vi "Trav_3D_volume.vi"(3 "Simulate/Run":T1, 5 "multirunIn":T2={"Start X"=0.0, "Start Y"=0.0, "Start Z"=0.0, "End X"=0.0, "End Y"=0.0, "End Z"=0.0, "nPoints"=0, "Spacing"=enum."Linear", "Filename"=path "", "Tunnel Speed"=0.0, "Averaging time (mins)"=0.0, "Extra Commands"="", "Carrier_1 Q (l/min)"=0.0, "Carrier_2 Q (l/min)"=0.0, "Trace Gas Concentration (%)"=0.0, "Specific Arguments"="", "Comments"="", "Row No"=0, "Row Type Selector"=enum."Traverse 3D Volume", "EstCompl"="", "Row Duration (mins)"=0.0, "nValidPoints"=0, "Meas Setup File"=""} {"Carrier_2 Q (l/min)" format="%#.2f"; "Row Duration (mins)" format="%#.1f"; "Row No" min=0; "Trace Gas Concentration (%)" min=0.0 format="%#_4f"; "Carrier_1 Q (l/min)" format="%#.4f"; "Start X" format="%#.2f"; "Start Y" format="%#.2f"; "Start Z" format="%#.2f"; "End X" format="%#.2f"; "End Y" format="%#.2f"; "End Z" format="%#.2f"; "Tunnel Speed" format="%#.2f"; "Averaging time (mins)" min=0.0 format="%#.2f"}) -> (0 "Error Messages":string, 1 "Status":T5, 2 "multirunOut":T2 {"Carrier_2 Q (l/min)" format="%#.2f"; "Row Duration (mins)" format="%#.1f"; "Row No" min=0; "Trace Gas Concentration (%)" min=0.0 format="%#_4f"; "Carrier_1 Q (l/min)" format="%#.4f"; "Start X" format="%#.2f"; "Start Y" format="%#.2f"; "Start Z" format="%#.2f"; "End X" format="%#.2f"; "End Y" format="%#.2f"; "End Z" format="%#.2f"; "Tunnel Speed" format="%#.2f"; "Averaging time (mins)" min=0.0 format="%#.2f"})   [LabVIEW 2021]
uses:
  Globals/Trav_pos_global.vi
  Globals/Meas_global.vi
  Controls/User_Specific_mode.ctl
  Gen Trav/Multi_Run_Status.ctl
  Controls/Setup.ctl
  Controls/Save_Data.ctl
  Controls/Overhead.ctl
  ADAM Client/Sub VIs/ADAM Controls/Traverse_Level_State.ctl
  Globals/Preference_global.vi
  Gen Trav/Spacing.ctl
  Gen Trav/Traverse_cluster.ctl
  Controls/Multi_run_mode.ctl
panel:
  in  "moveCostWeighting":sgl[](array[numeric])=[5.0, 2.0, 1.0]
  out "PredictedEnd":timestamp format="%<%H:%M\n%a %d>T"
  out "StartTime":timestamp format="%<%H:%M\n%a %d>T"
  out "Progress":i32(slide) scale=0.0..20.0
  in  "pointIDs":string[](array[string])
  in  "pointComments":string[](array[string])
  out "Pause message":string
  in  "Pause":bool
  out "Current position":dbl[](array[numeric]) format="%.2f"
  in  "stop":bool
  in  "Array of Positions":dbl[][](array[numeric]) format="%.2f"
  out "Abcissa copy":string="Y (mm)"
  out "Abcissa":string="Y (mm)"
  in  "Plot 1":i32[](listbox)=[1]
  out "U":cluster{dbl[], dbl[]}[](graph)
  out "% u'/U":cluster{dbl[], dbl[]}[](graph)
  # "Current Point"
  # "X           Y          Z"
  # "Start"
  # "End"
  # "X           Y          Z"
  # "Start"
  # "End"
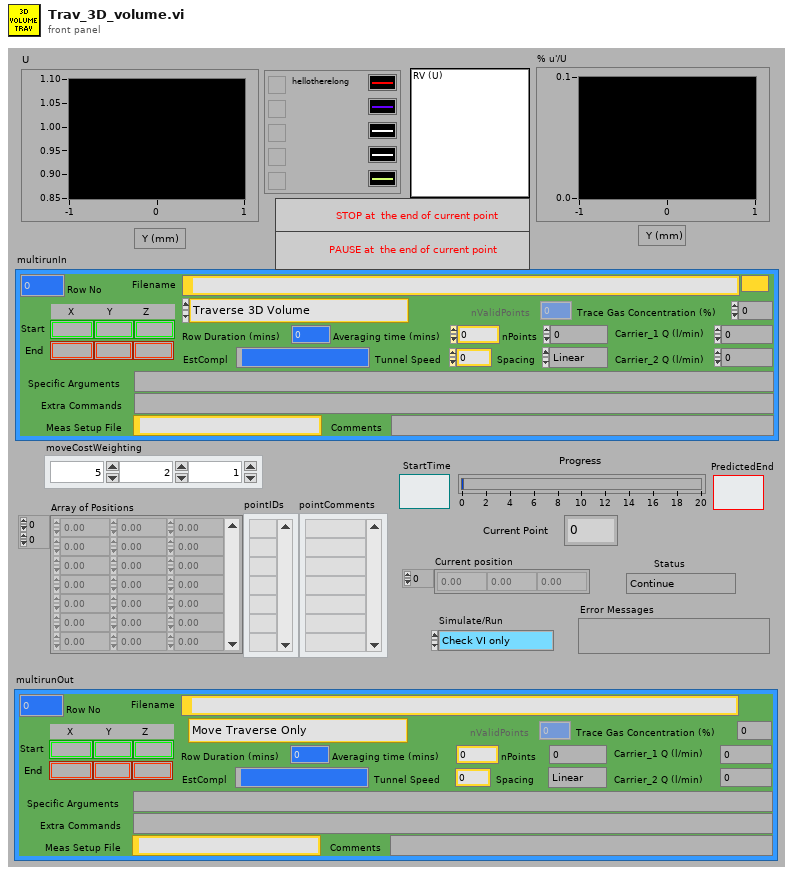
[diagram p1: front panel]
types:
  T1 = typedef "User_Specific_mode.ctl" = enum16{"Check VI only", "Run VI"}
  T2 = typedef "Traverse_cluster.ctl" = cluster{"Start X":sgl, "Start Y":sgl, "Start Z":sgl, "End X":sgl, "End Y":sgl, "End Z":sgl, "nPoints":i32, "Spacing":T3, "Filename":path, "Tunnel Speed":dbl, "Averaging time (mins)":dbl, "Extra Commands":string, "Carrier_1 Q (l/min)":dbl, "Carrier_2 Q (l/min)":dbl, "Trace Gas Concentration (%)":dbl, "Specific Arguments":string, "Comments":string, "Row No":i32, "Row Type Selector":T4, "EstCompl":string, "Row Duration (mins)":dbl, "nValidPoints":i32, "Meas Setup File":string}
  T3 = typedef "Spacing.ctl" = enum16{"Linear", "Log", "Gauss", "Specified", "N/A"}
  T4 = typedef "Multi_run_mode.ctl" = enum16{"Move Traverse Only", "Set Tunnel Speed Only", "Set Source Only", "Set Measurement Conditions", "Single Measurement", "Vertical Profile", "Lateral Profile", "Longitudinal Profile", "Multi-Axis Profile", "Explore Volume", "Auto Calibrate", "Meas Fast FID Bkgnd", "Check Beam Power", "Scanning Valve Measurement", "Run VI Named:", "Set ADAM Ch", "Wait (minutes)", "Send Message", "Synchronize With:", "Fall Back to this Row", "Turn Off Row Repeating", "Traverse 3D Volume", "Blank Row", "Jump to Fall Back Row"}
  T5 = typedef "Multi_Run_Status.ctl" = enum16{"Continue", "Continue with Error", "Jump to Next Point", "Jump to Next Row", "Jump To Fall Back", "Terminate Run"}
  T6 = typedef "Overhead.ctl" = enum16{"Update total times", "Read Current Overhead", "Re Scale totals to 3 hrs", "Initialise totals to 3hr"}
  T7 = typedef "Save_Data.ctl" = enum16{"Save No Data", "Save Data"}
  T8 = typedef "Setup.ctl" = enum16{"Run Program", "Show Setup", "Save Current Setup", "Setup Front Panel"}
  T9 = typedef "Traverse_Level_State.ctl" = enum16{"Running", "Complete"}
  T10 = typedef "GMU Gas Line Name.ctl" = enum16{"GMU1 Source", "GMU2 Source", "GMU2 Calib", "CPP GRC-A", "CPP GRC-B"}
  T11 = typedef "Status_Cluster.ctl" = cluster{"Status":T5, "Error Type":string, "Error Description":string}
  T12 = typedef "Analysis_info_cluster.ctl" = cluster{"Colour":u32, "Inst type":T13, "Inst name":string, "Symbol":string, "Code name":string, "Extra Info":string, "Inst Array":T14, "Extra Titles":string[], "Extra Values":string[], "U":dbl, "u^2":dbl, "u^3":dbl, "u^4":dbl, "Skew_u":dbl, "Kurt_u":dbl, "Sd Error in Mean":dbl, "% u'/U":dbl, "X":dbl, "Y":dbl, "Z":dbl, "Timescale integral Estimate":dbl, "Sd Error in Variance":dbl, "Calib File":path, "Calib Constants":dbl[], "Output Position":bool, "Stats":enum16{"None", "Basic", "Full"}, "Av Sampling Rate":dbl, "Av No of Samples":dbl, "Total Meas Time (s)":dbl, "ADAM Ch Name":string, "Max value":dbl, "Min value":dbl, "Req Sample Rate Hz":dbl, "Sync Delay Time (s)":dbl, "Ch No":i16, "Device":string, "Use Latest Calib":bool, "Port":string, "Metadata Ch Names":string[], "Metadata Ch Values":string[], "Label":string}
  T13 = typedef "Inst_type.ctl" = enum16{"Raw voltage", "Raw with zero offsetting", "Propeller anemometer", "Pressure Transducer", "Pitot-static tube", "Hot wire", "Cross wire 1", "Cross wire 2", "Generic Linear", "Generic Polynomial", "Generic BackPoly", "Fast FID", "Thermocouple", "Cold wire", "Pulsed Wire", "LDA Vel", "LDA Tran time", "LDA Arr time", "Microphone"}
  T14 = typedef "Instrument_Array.ctl" = enum16{"PWA", "LDA", "Analogue"}
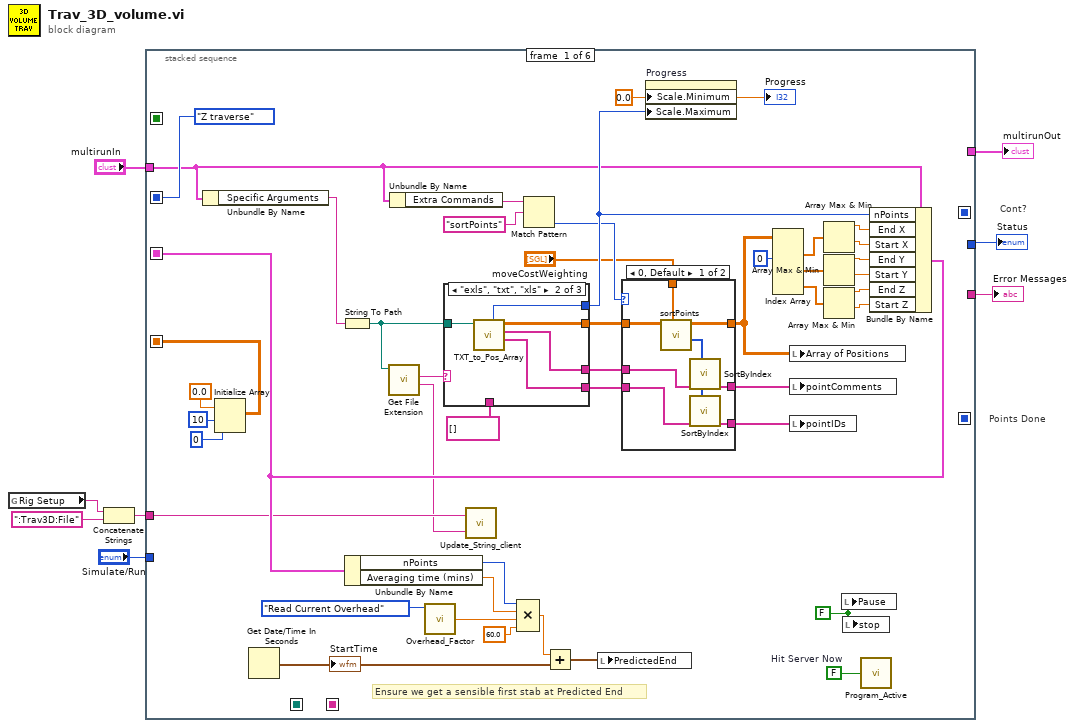
[diagram p0: block diagram]
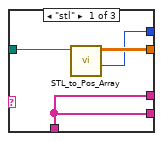
[diagram p3: hidden frame]
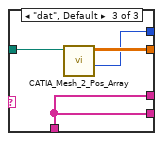
[diagram p4: hidden frame]
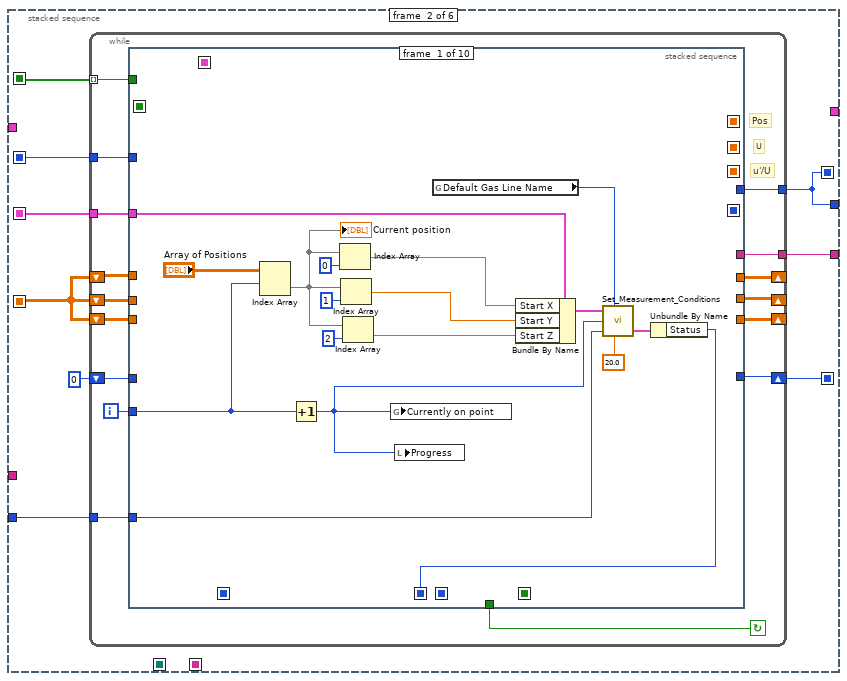
[diagram p5: hidden frame]
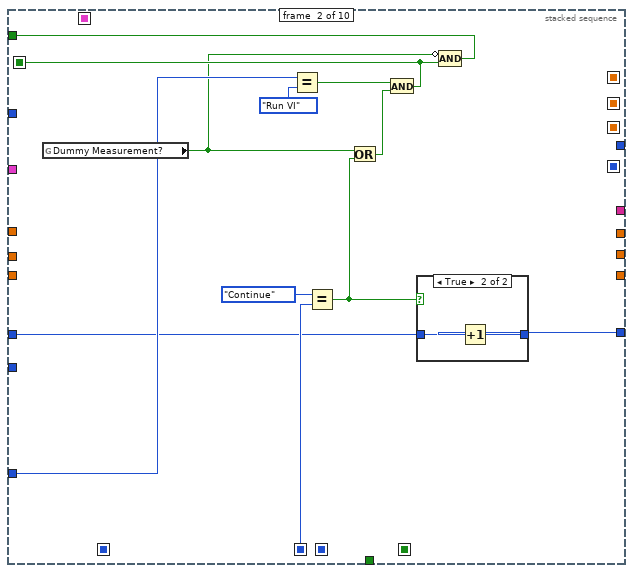
[diagram p6: hidden frame]
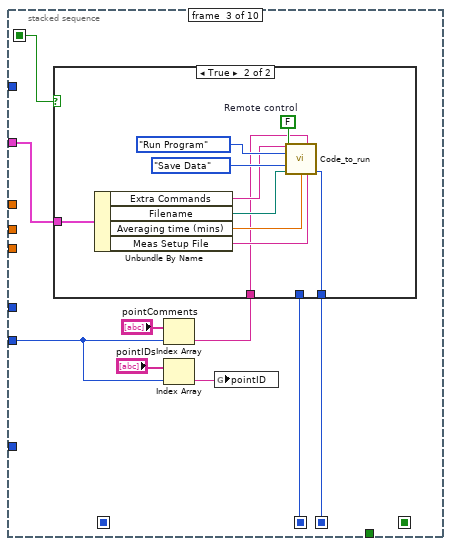
[diagram p8: hidden frame]
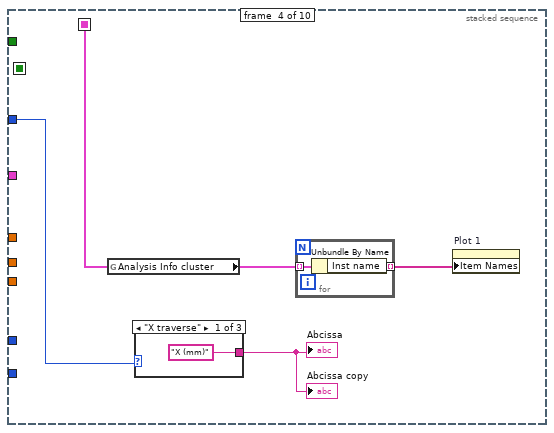
[diagram p10: hidden frame]
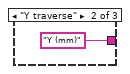
[diagram p11: hidden frame]
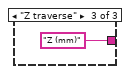
[diagram p12: hidden frame]
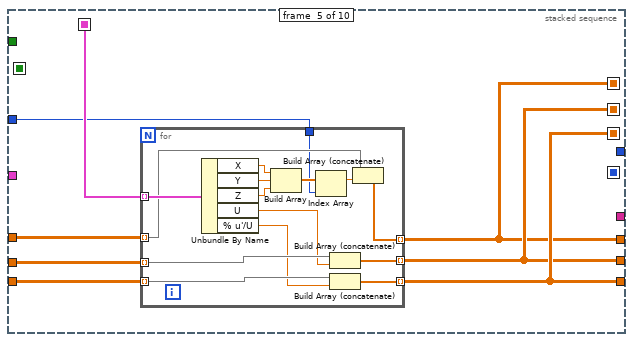
[diagram p13: hidden frame]
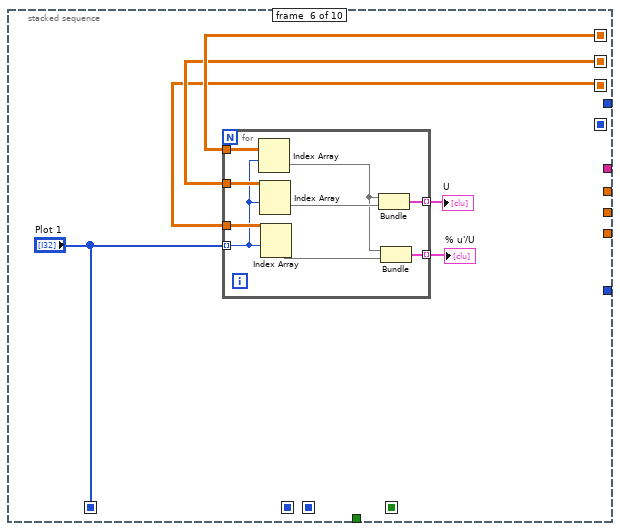
[diagram p14: hidden frame]
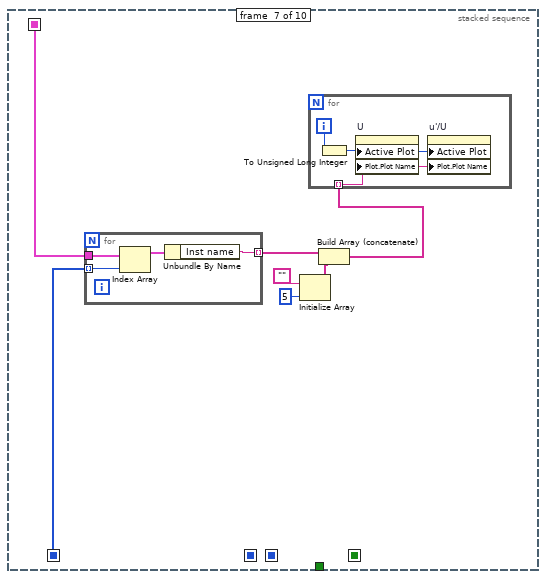
[diagram p15: hidden frame]
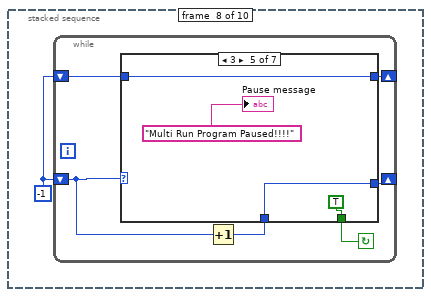
[diagram p16: hidden frame]
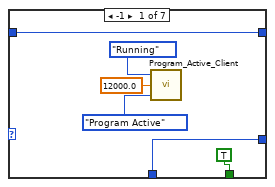
[diagram p17: hidden frame]
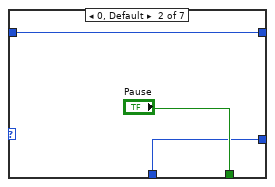
[diagram p18: hidden frame]
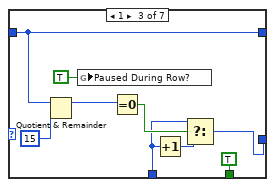
[diagram p19: hidden frame]
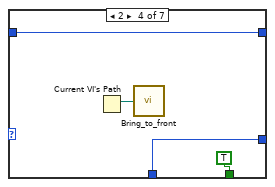
[diagram p20: hidden frame]
diagram:
  # "Points Done"
  # "Cont?"
  n1 = global read "Preference_global.vi" "Rig Setup"() -> (w4:string)
  n2 = Concatenate Strings(w4, ":Trav3D:File" ("string")) -> (w2:string)
  n3 = stacked-sequence {
    seq-local: [w50 _ _ _ _ _] -> [_ w85 _ _ _ _]
    seq-local: [enum16{"X traverse", "Y traverse", "Z traverse"}."Z traverse" ("Axis Traversed") _ _ _ _ _] -> [_ w86 _ _ _ _]
    seq-local: [_ _ w330 _ _ _] -> [_ _ _ _ w354 _]
    seq-local: [_ _ _ w337 _ _] -> [_ _ _ _ w353 _]
    seq-local: [_ w84 _ _ _ _] -> [_ _ _ _ _ _]
    seq-local: [_ w82 _ _ _ _] -> [_ _ _ w334 w352 _]
    seq-local: [_ w80 _ _ _ _] -> [_ _ _ _ _ w361]
    seq-local: [w30 _ _ _ _ _] -> [_ w79 _ _ _ w363]
    tunnel: [_ w84 _ _ _ _] -> w6
    tunnel: [_ _ _ _ _ w373] -> w8
    tunnel: "Simulate/Run" -> [_ w83 _ _ _ w372]
    tunnel: [_ w78 _ _ _ _] -> w5
    tunnel: w2 -> [w14 _ _ _ _ w360]
    tunnel: "multirunIn" -> [w10 _ _ _ _ _]
    frame #0 {
      w33 = 0.0 ("Data Entry Limits:Minimum")
      w48 = FALSE ("stop")
      w49 = FALSE  # Hit Server Now
      # "Ensure we get a sensible first stab at Predicted End"
      n4 = Unbundle By Name(w10) -> ("Specific Arguments"=w46:string)
      n5 = Initialize Array(0.0, 10, 0) -> (w50:dbl[][])
      n6 = Get Date/Time In Seconds() -> (seconds since 1Jan1904=w31:timestamp)
      "StartTime" <- w31
      n7 = String To Path(string=w46) -> (path=w13:path)
      n8 = call <vilib>:"Get File Extension.vi"("file"=w13) -> ("filename without extension"=w12:string, "lowercase file extension"=w11:string)  [unwired: 6 in, 3 out]
      n9 = Unbundle By Name(w10) -> ("Extra Commands"=w17:string)
      n10 = call "Overhead_Factor.vi"("Mode"=Overhead."Read Current Overhead") -> ("Current Overhead Factor"=w27:dbl)  [unwired: 3 in]
      n11 = case shown="\"exls\", \"txt\", \"xls\"" w11 {
        tunnel: [w67 w72 w77] -> w23
        tunnel: [w66 w70 w76] -> w34
        tunnel: w13 -> [w68 w73 w75]
        tunnel: [w65 w71 w74] -> w21
        tunnel: string[] [] ("pointComments") -> [w65 _ w74]
        tunnel: [w65 w69 w74] -> w19
        frame "stl" {
          n12 = call "STL_to_Pos_Array.vi"("STL file"=w68) -> ("Number of Points"=w66:i32, "Array of Positions"=w67:dbl[][])  [unwired: 9 in]
        }
        frame "exls", "txt", "xls" {
          n13 = call "TXT_to_Pos_Array.vi"("pointfile"=w73) -> ("pointIDs"=w69:string[], "pointComments"=w71:string[], "pointsXYZArray"=w72:dbl[][], "Number of Points"=w70:i32)  [unwired: 5 in, 2 out]
        }
        frame "dat", Default {
          n14 = call "CATIA_Mesh_2_Pos_Array.vi"("Catia Mesh File"=w75) -> ("Number of Points"=w76:i32, "Array of Positions"=w77:dbl[][])  [unwired: 9 in]
        }
      }
      n15 = call "Update_String_client.vi"("String"=w12, "Ch Name"=w14) -> ()  [unwired: 1 in]
      n16 = Match Pattern(string=w17, regular expression="sortPoints") -> (offset past match=w15:i32)  [unwired: 1 in, 3 out]
      n17 = case shown="0, Default" w15 {
        tunnel: w23 -> [w61 w64]
        tunnel: [w60 w64] -> w22
        tunnel: w21 -> [w59 w63]
        tunnel: [w58 w63] -> w20
        tunnel: w19 -> [w57 w62]
        tunnel: [w56 w62] -> w18
        tunnel: "moveCostWeighting" -> [w54 _]
        frame 0, Default {
          n18 = call "sortPoints.vi"("moveCostWeighting"=w54, "targetCoords"=w61) -> ("sortOrder"=w55:i32[], "sortedCoords"=w60:sgl[][])  [unwired: 8 in]
          n19 = call "SortByIndex.vi"("sortOrder"=w55, "1DstringIn"=w59) -> ("1DstringOut"=w58:string[])  [unwired: 4 in, 2 out]
          n20 = call "SortByIndex.vi"("sortOrder"=w55, "1DstringIn"=w57) -> ("1DstringOut"=w56:string[])  [unwired: 4 in, 2 out]
        }
        frame -1 {
        }
      }
      n21 = property on="Progress" class="Slide (strict)"("Scale.Minimum"=w33, "Scale.Maximum"=w34) -> ()  [unwired: 2 in, 2 out]
      n22 = Index Array(array=w22, index (col) #1=0 ("disabled index (col)")) -> (element #1=w43:dbl[], element #2=w40:dbl[], element #3=w35:dbl[])  [unwired: 5 in]
      n23 = local write "Array of Positions"(w22) -> ()
      n24 = local write "pointComments"(w20) -> ()
      n25 = local write "pointIDs"(w18) -> ()
      n26 = Array Max & Min(array=w43) -> (max value=w42:dbl, min value=w41:dbl)  [unwired: 2 out]
      n27 = Array Max & Min(array=w40) -> (max value=w39:dbl, min value=w38:dbl)  [unwired: 2 out]
      n28 = Array Max & Min(array=w35) -> (max value=w37:dbl, min value=w36:dbl)  [unwired: 2 out]
      n29 = local write "Pause"(w48) -> ()
      n30 = local write "stop"(w48) -> ()
      n31 = call "Program_Active.vi"("Hit Server Now"=w49) -> ()
      n32 = Bundle By Name(cluster=w10, "nPoints"=w34, "End X"=w42, "Start X"=w41, "End Y"=w39, "Start Y"=w38, "End Z"=w37, "Start Z"=w36) -> (w30:T2)
      n33 = Unbundle By Name(w30) -> ("nPoints"=w29:i32, "Averaging time (mins)"=w28:dbl)
      n34 = Compound Arithmetic op=MULTIPLY(w29, w28, w27, 60.0 ("value")) -> (w26:dbl)
      n35 = Add(x=w26, y=w31) -> (x+y=w25:timestamp)
      n36 = local write "PredictedEnd"(w25) -> ()
      "Progress" <- w33
    }
    frame #1 {
      n37 = while {
        shift-left: 0 -> [w89]
        shift-right: [w88] -> w80
        tunnel: [w90] -> w82 mode=indexing
        tunnel: w79 -> [w91]
        tunnel: w83 -> [w92]
        tunnel: [w93] -> w84
        shift-left: w85 -> [w96]
        shift-right: [w95] -> _
        tunnel: w86 -> [w97]
        shift-left: w85 -> [w99]
        shift-right: [w98] -> _
        shift-left: w85 -> [w101]
        shift-right: [w100] -> _
        tunnel: [w87] -> w78
        i -> [w102]
        stop <- w94 continue-if-true
        # "Pos"
        # "U"
        # "u'/U"
        n38 = stacked-sequence {
          seq-local: [_ _ _ w158 _ _ _ _ _ _] -> [_ _ _ _ w169 _ w202 _ _ _]
          seq-local: [_ _ _ _ w165 _ _ _ _ _] -> [_ _ _ _ _ w192 _ _ _ _]
          seq-local: [_ _ _ _ w167 _ _ _ _ _] -> [_ _ _ _ _ w191 _ _ _ _]
          seq-local: [_ _ _ _ w168 _ _ _ _ _] -> [_ _ _ _ _ w190 _ _ _ _]
          seq-local: [_ _ _ _ _ "Plot 1" _ _ _ _] -> [_ _ _ _ _ _ w208 _ _ _]
          seq-local: [_ _ w142 _ _ _ _ _ _ _] -> [_ _ _ _ _ _ _ _ w266 _]
          seq-local: [w109 _ _ _ _ _ _ _ _ _] -> [_ w129 w140 _ _ _ _ _ _ _]
          seq-local: [_ w122 _ _ _ _ _ _ _ _] -> [_ _ w141 _ _ _ _ _ _ _]
          seq-local: [_ _ _ _ _ _ _ _ w261 _] -> [_ _ _ _ _ _ _ _ _ w283]
          seq-local: [_ _ _ _ _ _ _ _ w260 _] -> [_ _ _ _ _ _ _ _ _ w277]
          tunnel: w102 -> [w107 _ w136 _ _ _ _ _ w272 w280]
          tunnel: w101 -> [_ _ _ _ w171 _ _ _ _ _]
          tunnel: [_ _ _ _ w167 _ _ _ _ _] -> w100
          tunnel: w99 -> [_ _ _ _ w170 _ _ _ _ _]
          tunnel: [_ _ _ _ w168 _ _ _ _ _] -> w98
          tunnel: w97 -> [_ _ _ w156 w164 _ _ _ _ _]
          tunnel: w96 -> [_ _ _ _ w166 _ _ _ _ _]
          tunnel: [_ _ _ _ w165 _ _ _ _ _] -> w95
          tunnel: [_ _ _ _ _ _ _ _ w261 _] -> w94
          tunnel: w91 -> [w113 _ w143 _ _ _ _ _ _ w281]
          tunnel: [_ _ _ _ _ _ _ _ _ w279] -> w93
          tunnel: w92 -> [w111 w131 _ _ _ _ _ _ _ w282]
          tunnel: [_ w121 _ _ _ _ _ _ _ _] -> w90
          tunnel: w89 -> [_ w126 _ _ _ _ _ _ _ w276]
          tunnel: [_ w125 _ _ _ _ _ _ _ _] -> w88
          tunnel: [_ _ _ _ _ _ _ _ _ w278] -> w87
          frame #0 {
            n39 = Index Array(array="Array of Positions", index (row)=w107) -> (element=w106:dbl[])  [unwired: 1 in]
            "Current position" <- w106
            n40 = Increment(x=w107) -> (x+1=w105:i32)
            n41 = Index Array(array=w106, index=0 ("Index")) -> (element=w116:dbl)
            n42 = Index Array(array=w106, index=1 ("Index")) -> (element=w115:dbl)
            n43 = Index Array(array=w106, index=2 ("Index")) -> (element=w114:dbl)
            n44 = global write "Trav_pos_global.vi" "Currently on point"(w105) -> ()
            n45 = local write "Progress"(w105) -> ()
            n46 = global read "Trav_pos_global.vi" "Default Gas Line Name"() -> (w104:T10)
            n47 = Bundle By Name(cluster=w113, "Start X"=w116, "Start Y"=w115, "Start Z"=w114) -> (w112:T2)
            n48 = call "Set_Measurement_Conditions.vi"("Traverse line"=w112, "Gas Line Name"=w104, "Currently on Point"=w105, "Simulate/Run"=w111, "Source Establishment Time (s)"=20.0) -> ("Status Cluster"=w110:T11)  [unwired: 2 in]
            n49 = Unbundle By Name(w110) -> ("Status"=w109:T5)
          }
          frame #1 {
            n50 = global read "Trav_pos_global.vi" "Dummy Measurement?"() -> (w120:bool)
            n51 = Equal?(x=w131, y=User_Specific_mode."Run VI" ("Simulate/Run")) -> (x = y?=w127:bool)
            n52 = Equal?(x=Multi_Run_Status."Continue" ("Status"), y=w129) -> (x = y?=w124:bool)
            n53 = Or(x=w120, y=w124) -> (x .or. y?=w123:bool)
            n54 = And(x=w127, y=w123) -> (x .and. y?=w122:bool)
            n55 = case shown="True" w124 {
              tunnel: w126 -> [w132 w134]
              tunnel: [w132 w133] -> w125
              frame False {
              }
              frame True {
                n56 = Increment(x=w134) -> (x+1=w133:i32)
              }
            }
            n57 = Compound Arithmetic op=AND(invert w120, w122) -> (w121:bool)
          }
          frame #2 {
            n58 = Index Array(array="pointComments", index=w136) -> (element=w138:string)
            n59 = case shown="True" w141 {
              tunnel: w143 -> [_ w154]
              tunnel: [w144 w153] -> w142
              tunnel: w140 -> [w144 _]
              tunnel: w138 -> [_ w145]
              frame False {
              }
              frame True {
                w152 = FALSE  # Remote control
                n60 = Unbundle By Name(w154) -> ("Extra Commands"=w146:string, "Filename"=w150:path, "Averaging time (mins)"=w151:dbl, "Meas Setup File"=w147:string)
                n61 = call "Code_to_run.vi"("Extra command String"=w146, "Current Row Comments"=w145, "setup"=Setup."Run Program", "Remote control"=w152, "File"=Save_Data."Save Data", "Results Filename"=w150, "Averaging time (min)"=w151, "Setup filename"=w147) -> ("Status"=w153:T5)  [unwired: 4 in, 3 out]
              }
            }
            n62 = Index Array(array="pointIDs", index=w136) -> (element=w135:string)
            n63 = global write "Trav_pos_global.vi" "pointID"(w135) -> ()
          }
          frame #3 {
            n64 = global read "Meas_global.vi" "Analysis Info cluster"() -> (w158:T12[])
            n65 = case shown="\"X traverse\"" w156 {
              tunnel: ["X (mm)" "Y (mm)" "Z (mm)"] -> w155
              frame "X traverse" {
              }
              frame "Y traverse" {
              }
              frame "Z traverse" {
              }
            }
            "Abcissa" <- w155
            "Abcissa copy" <- w155
            n66 = for {
              tunnel: w158 -> [w163] mode=indexing
              tunnel: [w162] -> w157 mode=indexing
              n67 = Unbundle By Name(w163) -> ("Inst name"=w162:string)
            }
            n68 = property on="Plot 1" class="LstBox (strict)"("Item Names"=w157) -> ()  [unwired: 2 in, 2 out]
          }
          frame #4 {
            n69 = for {
              tunnel: w171 -> [w186] mode=indexing
              tunnel: [w184] -> w167 mode=indexing
              tunnel: w170 -> [w183] mode=indexing
              tunnel: [w181] -> w168 mode=indexing
              tunnel: w169 -> [w180] mode=indexing
              tunnel: w166 -> [w179] mode=indexing
              tunnel: [w178] -> w165 mode=indexing
              tunnel: w164 -> [w173]
              n70 = Unbundle By Name(w180) -> ("X"=w177:dbl, "Y"=w176:dbl, "Z"=w175:dbl, "U"=w185:dbl, "% u'/U"=w182:dbl)
              n71 = Build Array(w177, w176, w175) -> (w174:dbl[])
              n72 = Index Array(array=w174, index=w173) -> (element=w172:dbl)
              n73 = Build Array (concatenate)(w186, w185) -> (w184:dbl[])
              n74 = Build Array (concatenate)(w183, w182) -> (w181:dbl[])
              n75 = Build Array (concatenate)(w179, w172) -> (w178:dbl[])
            }
          }
          frame #5 {
            n76 = for {
              tunnel: "Plot 1" -> [w193] mode=indexing
              tunnel: w192 -> [w201]
              tunnel: w191 -> [w200]
              tunnel: w190 -> [w199]
              tunnel: [w195] -> w189 mode=indexing
              tunnel: [w194] -> w188 mode=indexing
              n77 = Index Array(array=w201, index (row)=w193) -> (element=w197:dbl[])  [unwired: 1 in]
              n78 = Index Array(array=w200, index (row)=w193) -> (element=w198:dbl[])  [unwired: 1 in]
              n79 = Index Array(array=w199, index (row)=w193) -> (element=w196:dbl[])  [unwired: 1 in]
              n80 = Bundle(w197, w198) -> (w194:cluster{dbl[], dbl[]})  [unwired: 1 out]
              n81 = Bundle(w197, w196) -> (w195:cluster{dbl[], dbl[]})  [unwired: 1 out]
            }
            "U" <- w188
            "% u'/U" <- w189
          }
          frame #6 {
            n82 = for {
              tunnel: w208 -> [w212] mode=indexing
              tunnel: w202 -> [w210]
              tunnel: [w209] -> w205 mode=indexing
              n83 = Index Array(array=w210, index=w212) -> (element=w211:T12)
              n84 = Unbundle By Name(w211) -> ("Inst name"=w209:string)
            }
            n85 = Initialize Array("", 5) -> (w204:string[])
            n86 = Build Array (concatenate)(w205, w204) -> (w203:string[])
            n87 = for {
              tunnel: w203 -> [w213] mode=indexing
              i -> [w215]
              n88 = To Unsigned Long Integer(number=w215) -> (unsigned 32bit integer=w214:u32)
              n89 = property on="U" class="XYGraph (strict)"("Active Plot"=w214, "Plot.Plot Name"=w213) -> ()  [unwired: 2 in, 2 out]
              n90 = property on="u'/U" class="XYGraph (strict)"("Active Plot"=w214, "Plot.Plot Name"=w213) -> ()  [unwired: 2 in, 2 out]
            }
          }
          frame #7 {
            w216 = -1
            n91 = while {
              shift-left: w216 -> [w217]
              shift-right: [w218] -> _
              shift-left: w216 -> [w221]
              shift-right: [w222] -> _
              stop <- w219 continue-if-true
              n92 = Increment(x=w221) -> (x+1=w220:i32)
              n93 = case shown="3" w221 {
                tunnel: [w227 w230 w234 w244 w247 w251 0] -> w222
                tunnel: w220 -> [w227 w230 w236 w244 w247 w251 _]
                tunnel: [TRUE ("Pause") "Pause" TRUE ("Pause") TRUE ("Pause") TRUE ("Pause") TRUE ("Pause") TRUE ("Pause")] -> w219
                tunnel: [w226 w229 w232 w241 w245 w249 w254] -> w218
                tunnel: w217 -> [w226 w229 w232 w241 w245 w249 w255]
                frame -1 {
                  n94 = call "Program_Active_Client.vi"("Mode"=enum16{"Program Active", "Traverse Level State"}."Program Active", "Time till next contact (Sec)"=12000.0, "Traverse level State"=Traverse_Level_State."Running") -> ()  [unwired: 3 out]
                }
                frame 0, Default {
                }
                frame 1 {
                  n95 = Quotient & Remainder(x=w232, y=15) -> (x-y*floor(x/y)=w238:i32)  [unwired: 1 out]
                  n96 = global write "Trav_pos_global.vi" "Paused During Row?"(TRUE ("Paused During Row?")) -> ()
                  n97 = Equal To 0?(x=w238) -> (x = 0?=w237:bool)
                  n98 = Increment(x=w236) -> (x+1=w235:i32)
                  n99 = Select(t=w236, s=w237, f=w235) -> (s? t:f=w234:i32)
                }
                frame 2 {
                  n100 = Current VI's Path() -> (path=w242:path)
                  n101 = call "Bring_to_front.vi"("path"=w242) -> ()
                }
                frame 3 {
                  "Pause message" <- "Multi Run Program Paused!!!!" ("Pause message")
                }
                frame 4 {
                  n102 = property on="Pause message" class="Str"("Visible"=TRUE) -> ()  [unwired: 2 in, 2 out]
                  n103 = Wait Until Next ms Multiple(millisecond multiple=u32 1500) -> ()  [unwired: 1 out]
                }
                frame 5 {
                  n104 = Increment(x=w255) -> (x+1=w254:i32)
                  n105 = property on="Pause message" class="Str"("Visible"=FALSE) -> ()  [unwired: 2 in, 2 out]
                  n106 = Wait Until Next ms Multiple(millisecond multiple=u32 1500) -> ()  [unwired: 1 out]
                }
              }
            }
          }
          frame #8 {
            n107 = local read "Array of Positions"() -> (w262:dbl[][])
            n108 = Increment(x=w272) -> (x+1=w271:i32)
            n109 = Array Size(array=w262) -> (size(s)=w265:i32[])
            n110 = Index Array(array=w265, index=0 ("Index")) -> (element=w263:i32)
            n111 = case shown="\"Jump to Next Point\"" w266 {
              tunnel: [TRUE TRUE FALSE] -> w269
              frame "Continue" {
              }
              frame "Jump to Next Point" {
              }
              frame "Jump to Next Row", Default {
              }
            }
            n112 = Less?(x=w271, y=w263) -> (x < y?=w270:bool)
            n113 = Compound Arithmetic op=AND(w269, invert "stop", w270) -> (w261:bool)
            n114 = Select(t=Multi_Run_Status."Terminate Run" ("Status"), s="stop", f=w266) -> (s? t:f=w260:T5)
          }
          frame #9 {
            n115 = case shown="True" w283 {
              tunnel: w282 -> [_ w293]
              tunnel: w281 -> [_ w292]
              tunnel: w280 -> [_ w291]
              tunnel: [w285 w288] -> w279
              tunnel: ["" w287] -> w278
              tunnel: w277 -> [w285 _]
              tunnel: w276 -> [_ w286]
              frame False {
              }
              frame True {
                n116 = case shown="\"Check VI only\"" w293 {
                  tunnel: w292 -> [w309 w316]
                  tunnel: w291 -> [w304 _]
                  tunnel: [w294 timestamp(0 s since 1904-01-01)] -> w290
                  tunnel: w286 -> [_ w314]
                  frame "Check VI only" {
                    n117 = Increment(x=w304) -> (x+1=w302:i32)
                    n118 = Unbundle By Name(w309) -> ("Averaging time (mins)"=w306:dbl)
                    n119 = Multiply(x=60.0, y=w306) -> (x*y=w305:dbl)
                    n120 = Add(x=w305, y=10.0 ("Scalable Time (Sec)")) -> (x+y=w303:dbl)
                    n121 = global read "Trav_pos_global.vi" "Simulation Time"() -> (w296:timestamp)
                    n122 = Multiply(x=w303, y=w302) -> (x*y=w300:dbl)
                    n123 = call "Overhead_Factor.vi"("Mode"=Overhead."Read Current Overhead") -> ("Current Overhead Factor"=w301:dbl)  [unwired: 3 in]
                    n124 = To Double Precision Float(number=w296) -> (double precision float=w297:dbl)
                    n125 = Multiply(x=w301, y=w300) -> (x*y=w298:dbl)
                    n126 = Add(x=w297, y=w298) -> (x+y=w295:dbl)
                    n127 = To Time Stamp(1:w295) -> (0:w294:timestamp)
                  }
                  frame "Run VI" {
                    n128 = Unbundle By Name(w316) -> ("nValidPoints"=w315:i32)
                    n129 = local read "StartTime"() -> (w313:timestamp)
                    n130 = Get Date/Time In Seconds() -> (seconds since 1Jan1904=w317:timestamp)
                    n131 = Divide(x=w315, y=w314) -> (x/y=w312:dbl)
                    n132 = Subtract(x=w317, y=w313) -> (x-y=w311:dbl)
                    n133 = Multiply(x=w312, y=w311) -> (x*y=w310:dbl)
                    n134 = Add(x=w310, y=w313) -> (x+y=→"PredictedEnd":timestamp)
                  }
                }
                n135 = call "Run_FFID_Bkgnd.vi"("Simulated Time"=w290, "Run Now?"=FALSE, "Simulate/Run"=w293) -> ("Error Messages"=w287:string, "Status"=w288:T5)  [unwired: 1 out]
              }
            }
          }
        }
      }
    }
    frame #2 {
      n136 = global read "Meas_global.vi" "Start Time of experiment"() -> (w322:dbl)
      n137 = call "Sec_to_date_filename.vi"("ss1904"=w322) -> ("YYYY-mm-DD HH:MM"=w320:string)  [unwired: 5 in, 9 out]
      n138 = global read "Meas_global.vi" "Raw data file"() -> (w332:path)
      n139 = Format Into String(format string="Cmd_%s.xls", w320) -> (resulting string=w325:string)  [unwired: 2 in, 1 out]
      n140 = call "Fast_string_Replace.vi"("Replace match with:"="-", "Input String"=w325, "regular expression"=":") -> ("Output String"=w328:string)  [unwired: 2 out]
      n141 = Strip Path(path=w332) -> (stripped path=w331:path)  [unwired: 1 out]
      n142 = call "Fast_string_Replace.vi"("Replace match with:"="", "Input String"=w328, "regular expression"=" ") -> ("Output String"=w321:string)  [unwired: 2 out]
      n143 = Build Path(base path=w331, name or relative path=w321) -> (appended path=w330:path)
    }
    frame #3 {
      w343 = "\t"
      n144 = local read "Array of Positions"() -> (w336:dbl[][])
      n145 = Number To Fractional String(number=w336, precision (6)=i16 2) -> (F-format string=w335:string[][])  [unwired: 2 out]
      n146 = for {
        tunnel: w335 -> [w348] mode=indexing
        tunnel: w334 -> [w347] mode=indexing
        tunnel: [w345] -> w333 mode=indexing
        n147 = case shown="False" w347 {
          tunnel: ["Unobtainable Position" ""] -> w346
          frame False {
          }
          frame True {
          }
        }
        n148 = Build Array (concatenate)(w348, w346) -> (w345:string[])
      }
      n149 = Concatenate Strings("X", w343, "Y", w343, "Z") -> (w338:string)
      n150 = call "2D_array_to_string.vi"("2D data array"=w333, "Column titles  (separated by tabs)"=w338, "Array title"="Requested positions") -> ("Output string"=w337:string)
    }
    frame #4 {
      n151 = Or Array Elements(Boolean array=w352) -> (logical OR=w351:bool)
      n152 = case shown="True" w351 {
        tunnel: w354 -> [_ w357]
        tunnel: w353 -> [_ w355]
        frame False {
        }
        frame True {
          w356 = FALSE  # Lock File
          w358 = TRUE  # append to file? (new file:F)
          n153 = call "Write_Characters_To_File.vi"("file path (dialog if empty)"=w357, "character string"=w355, "append to file? (new file:F)"=w358, "Lock File"=w356) -> ()  [unwired: 1 in, 4 out]
        }
      }
    }
    frame #5 {
      n154 = local read "Array of Positions"() -> (w365:dbl[][])
      n155 = Array Size(array=w365) -> (size(s)=w367:i32[])
      n156 = Index Array(array=w367, index=0 ("Index")) -> (element=w364:i32)
      n157 = Bundle By Name(cluster=w363, "nValidPoints"=w361) -> (w362:T2)
      n158 = Not Equal?(x=w364, y=w361) -> (x != y?=w370:bool)
      n159 = Equal?(x=User_Specific_mode."Run VI" ("Simulate/Run"), y=w372) -> (x = y?=w369:bool)
      n160 = And(x=w369, y=w370) -> (x .and. y?=w368:bool)
      n161 = call "Update_String_client.vi"("String"="", "Ch Name"=w360) -> ()  [unwired: 1 in]
      n162 = case shown="True" w368 {
        tunnel: w362 -> [w374 w386]
        tunnel: [w374 w385] -> w373
        tunnel: w361 -> [_ w384]
        frame False {
        }
        frame True {
          w375 = " !!Program added comments"
          n163 = Unbundle By Name(w386) -> ("Comments"=w376:string)
          n164 = Equal To 0?(x=w384) -> (x = 0?=w383:bool)
          n165 = Match Pattern(string=w376, regular expression=w375) -> (match substring=w378:string)  [unwired: 4 out]
          n166 = Select(t=" !!(Row Skipped)", s=w383, f=" !!(Row Partially Skipped)") -> (s? t:f=w379:string)
          n167 = Empty String/Path?(string/path=w378) -> (empty?=w377:bool)
          n168 = case shown="True" w377 {
            tunnel: [w389 w393] -> w380
            tunnel: w379 -> [w388 w392]
            tunnel: w375 -> [_ w391]
            tunnel: w376 -> [w387 w390]
            frame False {
              n169 = Concatenate Strings(w387, w388) -> (w389:string)
            }
            frame True {
              n170 = Concatenate Strings(w390, w391, w392) -> (w393:string)
            }
          }
          n171 = Bundle By Name(cluster=w386, "Comments"=w380) -> (w385:T2)
        }
      }
    }
  }
  "Status" <- w6
  "multirunOut" <- w8
  "Error Messages" <- w5
